vi "Tração Torig e Tmax.vi"(8 "error in (no error)":errorcluster, 11 "Dados SP":T1={"Condutor"={"Pc (N/m)"=0.0, "Mod.Young (N/m²)"=0.0, "Dil.Term.c (m/°C)"=0.0, "Área  (m²)"=0.0, "Tração EDS (N)"=0.0, "Tração Torig(N)"=0.0, "Tração Talta (N)"=0.0}, "Suporte"={"Ps (N/m)"=0.0, "Es (N/m²)"=0.0, "DTc (1/°C)"=0.0, "Área sup (m²)"=0.0, "Tração EDS sup (N)"=0.0, "Tração AT sup (N)"=0.0, "Flecha sup AT (m)"=0.0}, "Projeto"={"Temp. EDS (°C)"=0.0, "Lim.original (°C)"=0.0, "Lim.extend. (°C)"=0.0, "N. cabo/fase"=1.0}, "Vetor de dados"={"Coor.X.esp"=[], "Coor.Y.Esp."=[], "Sub.vao X"=[], "Sub.vao Y"=[], "CoordY.sup"=[], "CoordX.sup"=[]}, "Subvão"={"N. Esp."=0.0, "F.lim (m)"=0.0, "Ext.calc"=0.0, "Ext.definido"=0.0, "Comp.cabo"=0.0, "Ext.55%"=0.0, "Tração sub\nAT (N)"=0.0, "Ext.sel."=0.0, "Flecha lim.\ncalc (m)"=0.0}, "Vão"={"Extensão (m)"=0.0, "Desnivel (m)"=0.0, "Ext.Lim sub (m)"=0.0, "Flecha à 60 °C"=0.0}} {"Projeto"."N. cabo/fase" min=1.0 max=8.0 step=1.0 format="%#_1f"}) -> (0 "error out":errorcluster, 3 "Dados SP Out":T1={"Condutor"={"Pc (N/m)"=0.0, "Mod.Young (N/m²)"=0.0, "Dil.Term.c (m/°C)"=0.0, "Área  (m²)"=0.0, "Tração EDS (N)"=0.0, "Tração Torig(N)"=0.0, "Tração Talta (N)"=0.0}, "Suporte"={"Ps (N/m)"=0.0, "Es (N/m²)"=0.0, "DTc (1/°C)"=0.0, "Área sup (m²)"=0.0, "Tração EDS sup (N)"=0.0, "Tração AT sup (N)"=0.0, "Flecha sup AT (m)"=0.0}, "Projeto"={"Temp. EDS (°C)"=0.0, "Lim.original (°C)"=0.0, "Lim.extend. (°C)"=0.0, "N. cabo/fase"=1.0}, "Vetor de dados"={"Coor.X.esp"=[], "Coor.Y.Esp."=[], "Sub.vao X"=[], "Sub.vao Y"=[], "CoordY.sup"=[], "CoordX.sup"=[]}, "Subvão"={"N. Esp."=0.0, "F.lim (m)"=0.0, "Ext.calc"=0.0, "Ext.definido"=0.0, "Comp.cabo"=0.0, "Ext.55%"=0.0, "Tração sub\nAT (N)"=0.0, "Ext.sel."=0.0, "Flecha lim.\ncalc (m)"=0.0}, "Vão"={"Extensão (m)"=0.0, "Desnivel (m)"=0.0, "Ext.Lim sub (m)"=0.0, "Flecha à 60 °C"=0.0}} {"Projeto"."N. cabo/fase" min=1.0 max=8.0 step=1.0 format="%#_1f"})   [LabVIEW 2020]
uses:
  controles/SP data.ctl
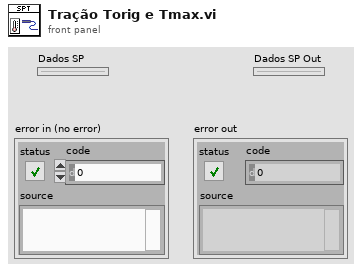
[diagram p1: front panel]
types:
  T1 = typedef "SP data.ctl" = cluster{"Condutor":cluster{"Pc (N/m)":dbl, "Mod.Young (N/m²)":dbl, "Dil.Term.c (m/°C)":dbl, "Área  (m²)":dbl, "Tração EDS (N)":dbl, "Tração Torig(N)":dbl, "Tração Talta (N)":dbl}, "Suporte":cluster{"Ps (N/m)":dbl, "Es (N/m²)":dbl, "DTc (1/°C)":dbl, "Área sup (m²)":dbl, "Tração EDS sup (N)":dbl, "Tração AT sup (N)":dbl, "Flecha sup AT (m)":dbl}, "Projeto":cluster{"Temp. EDS (°C)":dbl, "Lim.original (°C)":dbl, "Lim.extend. (°C)":dbl, "N. cabo/fase":dbl}, "Vetor de dados":cluster{"Coor.X.esp":dbl[], "Coor.Y.Esp.":dbl[], "Sub.vao X":dbl[], "Sub.vao Y":dbl[], "CoordY.sup":dbl[], "CoordX.sup":dbl[]}, "Subvão":cluster{"N. Esp.":dbl, "F.lim (m)":dbl, "Ext.calc":dbl, "Ext.definido":dbl, "Comp.cabo":dbl, "Ext.55%":dbl, "Tração sub\nAT (N)":dbl, "Ext.sel.":dbl, "Flecha lim.\ncalc (m)":dbl}, "Vão":cluster{"Extensão (m)":dbl, "Desnivel (m)":dbl, "Ext.Lim sub (m)":dbl, "Flecha à 60 °C":dbl}}
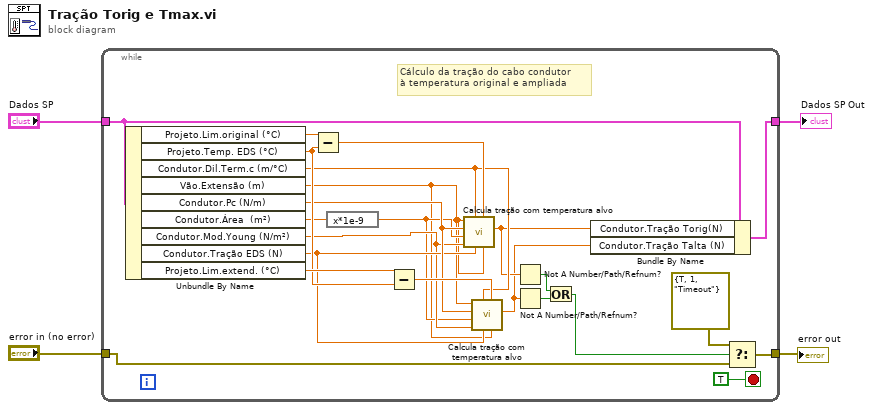
[diagram p0: block diagram]
diagram:
  n1 = while {
    tunnel: "Dados SP" -> [w25]
    tunnel: [w24] -> w3
    tunnel: [w6] -> w1
    tunnel: "error in (no error)" -> [w7]
    stop <- TRUE stop-if-true
    # "Cálculo da tração do cabo condutor\nà temperatura original e ampliada"
    n2 = Unbundle By Name(w25) -> ("Projeto.Lim.original (°C)"=w22:dbl, "Projeto.Temp. EDS (°C)"=w21:dbl, "Condutor.Dil.Term.c (m/°C)"=w19:dbl, "Vão.Extensão (m)"=w13:dbl, "Condutor.Pc (N/m)"=w18:dbl, "Condutor.Área  (m²)"=w17:dbl, "Condutor.Mod.Young (N/m²)"=w15:dbl, "Condutor.Tração EDS (N)"=w16:dbl, "Projeto.Lim.extend. (°C)"=w23:dbl)
    n3 = Subtract(x=w22, y=w21) -> (x-y=w27:dbl)
    n4 = expression code="x*1e-9"(w17) -> (w14:dbl)
    n5 = Subtract(x=w23, y=w21) -> (x-y=w20:dbl)
    n6 = call "Calcula tração com temperatura alvo.vi"("A1 (m)"=w13, "t2-t1 (°C)"=w27, "To1 (N)"=w16, "Alfa t (1/°C)"=w19, "E (Pa)"=w15, "S (m²)"=w14, "p (N/m)"=w18, "Ao (m)"=w13) -> ("To2 Real  (N)"=w12:dbl)  [unwired: 3 in]
    n7 = call "Calcula tração com temperatura alvo.vi"("A1 (m)"=w13, "t2-t1 (°C)"=w20, "To1 (N)"=w16, "Alfa t (1/°C)"=w19, "E (Pa)"=w15, "S (m²)"=w14, "p (N/m)"=w18, "Ao (m)"=w13) -> ("To2 Real  (N)"=w11:dbl)  [unwired: 3 in]
    n8 = Not A Number/Path/Refnum?(number/path/refnum=w12) -> (NaN/Path/Refnum?=w9:bool)
    n9 = Not A Number/Path/Refnum?(number/path/refnum=w11) -> (NaN/Path/Refnum?=w10:bool)
    n10 = Or(x=w9, y=w10) -> (x .or. y?=w8:bool)
    n11 = Bundle By Name(cluster=w25, "Condutor.Tração Torig(N)"=w12, "Condutor.Tração Talta (N)"=w11) -> (w24:T1)
    n12 = Select(t=errorcluster {"status"=TRUE, "code"=1, "source"="Timeout"}, s=w8, f=w7) -> (s? t:f=w6:errorcluster)
  }
  "Dados SP Out" <- w3
  "error out" <- w1
